vi "channel names (units).vi"(5 "Sensor Array":T1) -> (2 "channel strings":string[](array[string]))   [LabVIEW 2012]
uses:
  DAQ configuration/Sensor array.ctl
  DAQ configuration/channel identifier.ctl
  calibration/global scale array.vi
  DataServer/Server Stats.vi
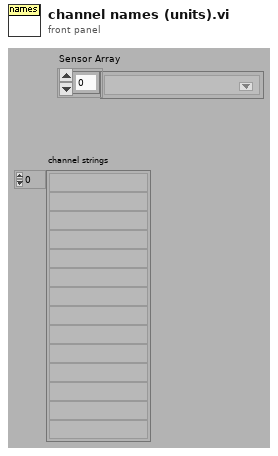
[diagram p1: front panel]
types:
  T1 = typedef "Sensor array.ctl" = T2[]
  T2 = typedef "channel identifier.ctl" = u16
  T3 = typedef "calib array.ctl" = T4[]
  T4 = typedef "conversion.ctl" = cluster{"conversion matrix":sgl[][], "units":string, "name":string, "scale type":T5, "offset (volts)":dbl, "second channel":i8, "correspondence table":T6, "offset (physical units)":dbl, "pH scale":T7, "D.O.":T8}
  T5 = typedef "scale type.ctl" = enum16{"Volts", "Polynomial", "Correspondence Table", "pH", "Dissolved Oxygen", "Quadratic"}
  T6 = typedef "correspondence table.ctl" = cluster{"physical units":dbl, "volts":dbl}[]
  T7 = typedef "pH scale.ctl" = cluster{"Buffers":cluster{"Buffer":dbl, "Calibrated":bool, "V/T":dbl}[], "Temperature":dbl}
  T8 = typedef "DO scale.ctl" = cluster{"Temperature":dbl, "K":dbl, "barometric pressure":dbl}
  T9 = typedef "Server stats.ctl" = cluster{"scan rate":dbl, "# connections":i32, "channel settings":cluster{"Name":string, "upper input limits":sgl, "lower input limits":sgl, "Location":string}[]}
  T10 = cluster{"Name":string, "upper input limits":sgl, "lower input limits":sgl, "Location":string}[]
  T11 = cluster{"Name":string, "upper input limits":sgl, "lower input limits":sgl, "Location":string}
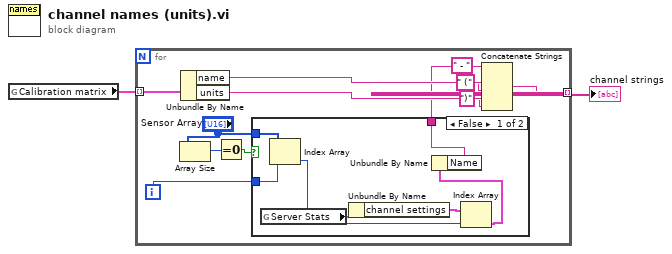
[diagram p0: block diagram]
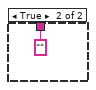
[diagram p2: hidden frame]
diagram:
  n1 = global read "global scale array.vi" "Calibration matrix"() -> (w2:T3)
  n2 = for {
    tunnel: w2 -> [w14] mode=indexing
    tunnel: [w9] -> w1 mode=indexing
    i -> [w5]
    n3 = Array Size(array="Sensor Array") -> (size(s)=w6:i32)
    n4 = Unbundle By Name(w14) -> ("name"=w13:string, "units"=w11:string)
    n5 = Equal To 0?(x=w6) -> (x = 0?=w7:bool)
    n6 = case shown="False" w7 {
      tunnel: w5 -> [w21 _]
      tunnel: "Sensor Array" -> [w20 _]
      tunnel: [w15 ""] -> w4
      frame False {
        n7 = global read "Server Stats.vi" "Server Stats"() -> (w19:T9)
        n8 = Index Array(array=w20, index=w21) -> (element=w17:T2)
        n9 = Unbundle By Name(w19) -> ("channel settings"=w18:T10)
        n10 = Index Array(array=w18, index=w17) -> (element=w16:T11)
        n11 = Unbundle By Name(w16) -> ("Name"=w15:string)
      }
      frame True {
      }
    }
    n12 = Concatenate Strings(w4, " - " ("string"), w13, " (" ("Substring"), w11, ")" ("Substring")) -> (w9:string)
  }
  "channel strings" <- w1
